vi "Sequence.Build.vi"(8 "error in (no error)":errorcluster, 11 "State Variables":T1={"Aliases.All"=[], "Aliases.Outputs"=[], "UI.Sequence#ofColumns"=0, "SysDef.Path"=path "", "UI.SequenceRef"=refnum, "UI.StepInformationRef"=refnum, "UI.AbortRef"=refnum, "UI.GraphRef"=refnum, "UI.ViewRef"=refnum, "UI.IterationsRef"=refnum, "UI.IterationInformationRef"=refnum, "INI.Settings"={"Build Location"=path "C:/Simple Sequence Editor/SequenceRepo", "LoggingLocation"=path ""}, "NIVS.Workspace Event"=refnum, "UI.SkipChannel"=refnum, "NIVS.Launched?"=FALSE, "UI.DurationChannel"=refnum}) -> (0 "error out":errorcluster)   [LabVIEW 2015, in "Simple Sequence Tools - Editor.lvlib"]
uses:
  Simple Sequence Tools - Editor.lvlib
  Types/Main.StateVariables.ctl
  Shared/Types/Channel.Properties.ctl
  Shared/Types/INI.Settings.ctl
  Shared/Simple Sequence Tools - Shared.lvlib
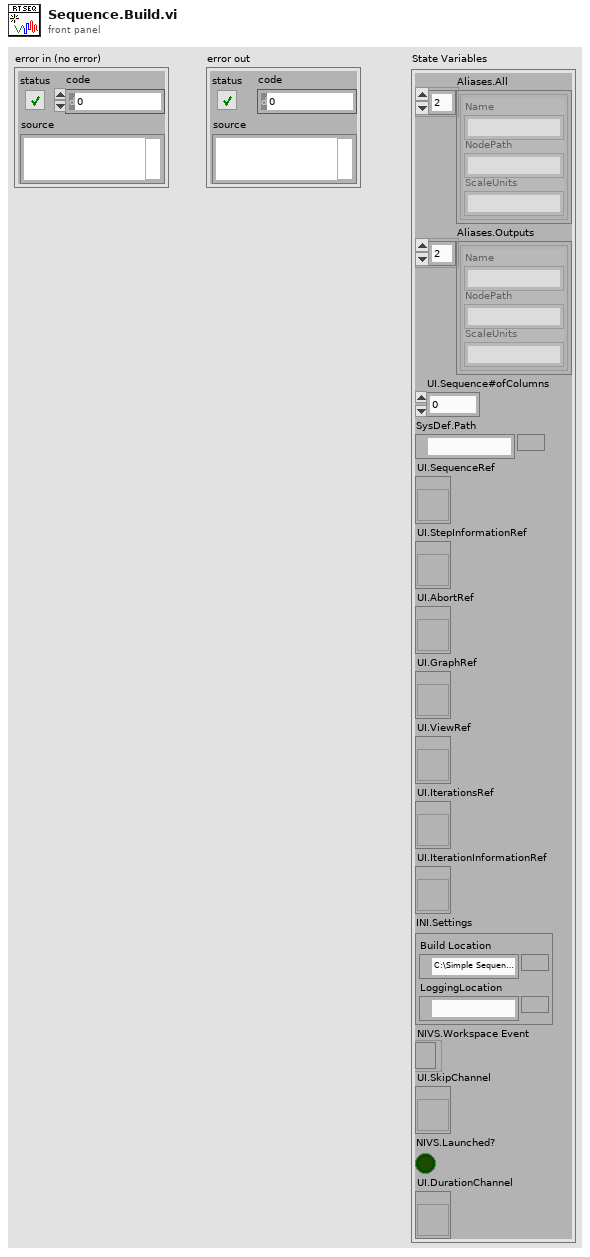
[diagram p1: front panel]
types:
  T1 = typedef "Simple Sequence Tools - Editor.lvlib/Main.StateVariables.ctl" = cluster{"Aliases.All":T2[], "Aliases.Outputs":T2[], "UI.Sequence#ofColumns":i32, "SysDef.Path":path, "UI.SequenceRef":refnum<vi>, "UI.StepInformationRef":refnum<vi>, "UI.AbortRef":refnum<vi>, "UI.GraphRef":refnum<vi>, "UI.ViewRef":refnum<vi>, "UI.IterationsRef":refnum<vi>, "UI.IterationInformationRef":refnum<vi>, "INI.Settings":T3, "NIVS.Workspace Event":refnum<event-registration>, "UI.SkipChannel":refnum<vi>, "NIVS.Launched?":bool, "UI.DurationChannel":refnum<vi>}
  T2 = typedef "Simple Sequence Tools - Shared.lvlib/Channel.Properties.ctl" = cluster{"Name":string, "NodePath":string, "ScaleUnits":string}
  T3 = typedef "Simple Sequence Tools - Shared.lvlib/INI.Settings.ctl" = cluster{"Build Location":path, "LoggingLocation":path}
  T4 = typedef "Simple Sequence Tools - Editor.lvlib/Compiled.RTSequenceProperties.ctl" = cluster{"Channels":T2[], "Steps":T5[], "Iterations":u32, "Sequence Channels":T11}
  T5 = typedef "Simple Sequence Tools - Editor.lvlib/Compiled.StepProperties.ctl" = cluster{"IOState":T6, "Condition":T9}
  T6 = typedef "Simple Sequence Tools - Editor.lvlib/Compiled.IOStateProperties.ctl" = cluster{"Duration":dbl, "Elements":T7[]}
  T7 = typedef "Simple Sequence Tools - Editor.lvlib/Compiled.StepElementProperties.ctl" = cluster{"Channel":T2, "Step":T8, "Parameters":dbl[]}
  T8 = typedef "Simple Sequence Tools - Shared.lvlib/Step.Types.ctl" = enum8{"Step", "iStep", "Ramp", "Unchanged", "Unknown", "Sine", "LogSine", "LinearSine", "ForcedRamp", "SquareWave"}
  T9 = typedef "Simple Sequence Tools - Editor.lvlib/Compiled.StepCondition.ctl" = cluster{"First Opreation":T10, "Expression":string}
  T10 = typedef "Simple Sequence Tools - Editor.lvlib/Conditions.OperationTypes.ctl" = enum8{"None", "&&", "||"}
  T11 = typedef "Simple Sequence Tools - Editor.lvlib/Compiled.SequenceChannels.ctl" = cluster{"Abort":T2, "IterationInfo":T2, "StepInfo":T2, "Skip":T2, "Duration":T2}
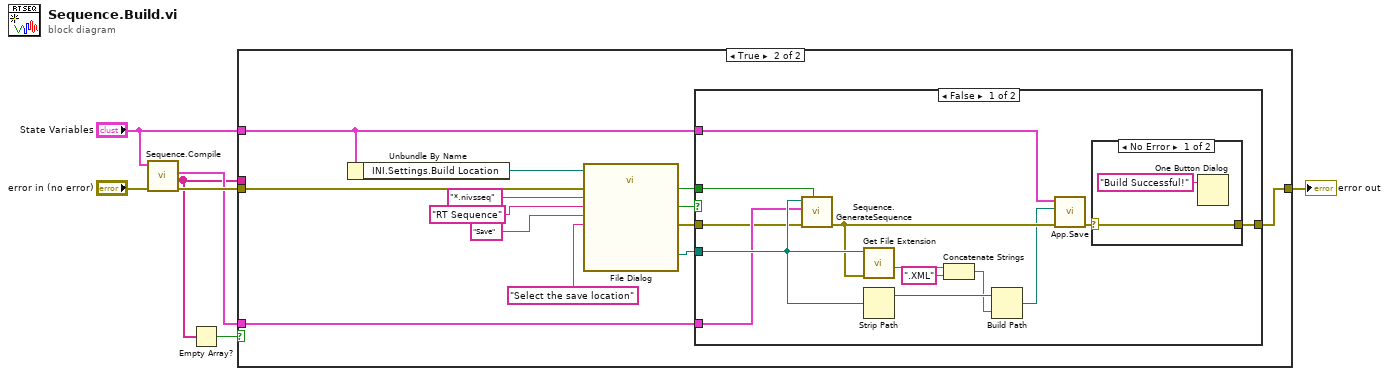
[diagram p0: block diagram]
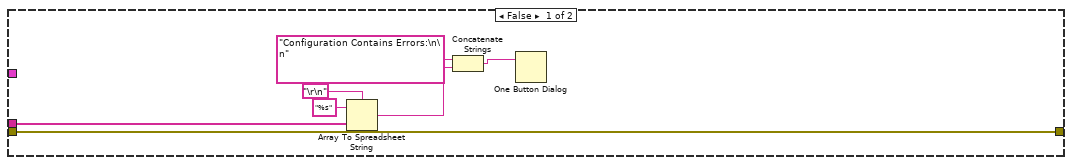
[diagram p2: hidden frame]
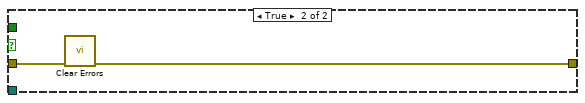
[diagram p4: hidden frame]
diagram:
  n1 = call "Sequence.Compile.vi"("error in (no error)"="error in (no error)", "State Variables"="State Variables") -> ("error out"=w5:errorcluster, "Warnings"=w1:string[], "CompiledSettings"=w4:T4)  [unwired: 7 in]
  n2 = Empty Array?(array=w1) -> (empty?=w2:bool)
  n3 = case shown="True" w2 {
    tunnel: [w14 w20] -> w7
    tunnel: w5 -> [w14 w17]
    tunnel: w4 -> [_ w19]
    tunnel: "State Variables" -> [_ w18]
    tunnel: w1 -> [w12 _]
    frame False {
      n4 = Array To Spreadsheet String(delimiter (Tab)="\r\n", array=w12, 3:"%s" ("format string")) -> (spreadsheet string=w10:string)
      n5 = Concatenate Strings("Configuration Contains Errors:\n\n", w10) -> (w13:string)
      n6 = One Button Dialog(message=w13) -> ()  [unwired: 1 in, 1 out]
    }
    frame True {
      n7 = Unbundle By Name(w18) -> ("INI.Settings.Build Location"=w16:path)
      n8 = call "File Dialog"("start path"=w16, "prompt"="Select the save location", "button label"="Save", "error in"=w17, "pattern (all files)"="*.nivsseq", "pattern label"="RT Sequence") -> ("selected path"=w25:path, "exists"=w15:bool, "cancelled"=w26:bool, "error out"=w27:errorcluster)  [unwired: 6 in]
      n9 = case shown="False" w26 {
        tunnel: [w29 w44] -> w20
        tunnel: w27 -> [w32 w45]
        tunnel: w25 -> [w40 _]
        tunnel: w19 -> [w33 _]
        tunnel: w18 -> [w31 _]
        tunnel: w15 -> [w28 _]
        frame False {
          n10 = call "Sequence.GenerateSequence.vi"("Exists"=w28, "error in (no error)"=w32, "Compiled Settings"=w33, "Path"=w40) -> ("error out"=w39:errorcluster)  [unwired: 7 in]
          n11 = call <vilib>:"Get File Extension.vi"("error in (no error)"=w39, "file"=w40) -> ("filename without extension"=w37:string)  [unwired: 5 in, 4 out]
          n12 = Strip Path(path=w40) -> (stripped path=w38:path)  [unwired: 1 out]
          n13 = Concatenate Strings(w37, ".XML" ("string")) -> (w35:string)
          n14 = Build Path(base path=w38, name or relative path=w35) -> (appended path=w34:path)
          n15 = call "App.Save.vi"("error in (no error)"=w39, "selected path"=w34, "State Variables"=w31) -> ("error out"=w30:errorcluster)  [unwired: 8 in]
          n16 = case shown="No Error" w30 {
            selector: w30 -> [w42 w43]
            tunnel: [w42 w43] -> w29
            frame No Error {
              n17 = One Button Dialog(message="Build Successful!") -> ()  [unwired: 1 in, 1 out]
            }
            frame Error {
            }
          }
        }
        frame True {
          n18 = call <vilib>:"Clear Errors.vi"("error in (no error)"=w45) -> ("error out"=w44:errorcluster)  [unwired: 5 in, 1 out]
        }
      }
    }
  }
  "error out" <- w7
